vi "Init Edge Detection.vi"(6 "Unsee last word":bool=TRUE, 8 "error in (no error)":errorcluster, 9 "Last output":dbl, 10 "First output":dbl, 11 "RP Transceiver in":refnum<class "RP Transceiver.lvclass">) -> (0 "error out":errorcluster, 3 "RP Transceiver out":refnum<class "RP Transceiver.lvclass">)   [LabVIEW 2016, in "RP Transceiver.lvclass"]
uses:
  RP Transceiver.lvclass
  RP Transceiver.lvclass/RP Transceiver.ctl
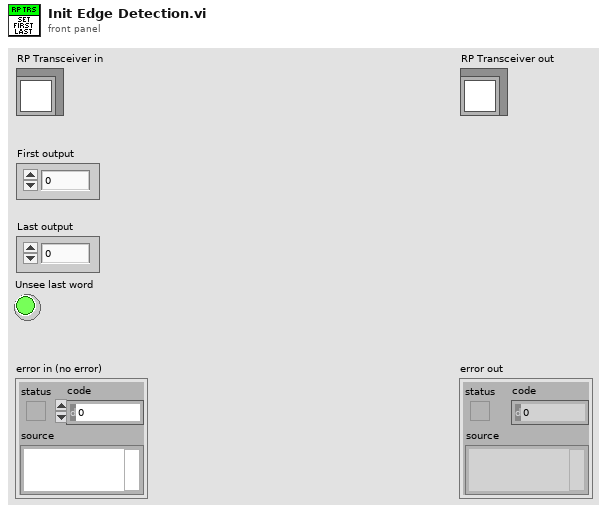
[diagram p1: front panel]
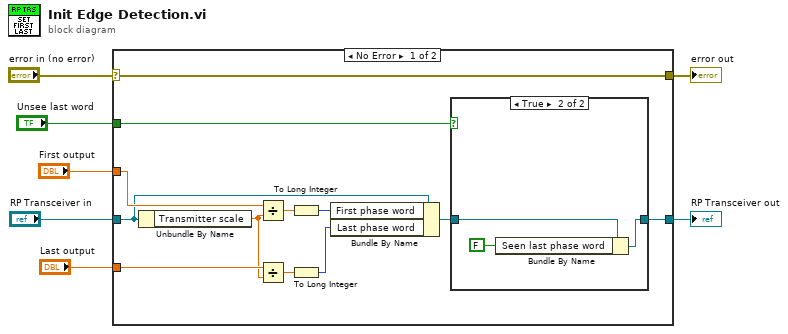
[diagram p0: block diagram]
diagram:
  n1 = case shown="No Error" "error in (no error)" {
    selector: "error in (no error)" -> [w19 w25]
    tunnel: [w19 w25] -> w6
    tunnel: [w9 w24] -> w4
    tunnel: "RP Transceiver in" -> [w11 w24]
    tunnel: "First output" -> [w18 _]
    tunnel: "Last output" -> [w17 _]
    tunnel: "Unsee last word" -> [w8 _]
    frame No Error {
      n2 = Unbundle By Name(w11) -> ("Transmitter scale"=w16:dbl)
      n3 = Divide(x=w18, y=w16) -> (x/y=w15:dbl)
      n4 = Divide(x=w17, y=w16) -> (x/y=w14:dbl)
      n5 = To Long Integer(number=w15) -> (32bit integer=w13:i32)
      n6 = To Long Integer(number=w14) -> (32bit integer=w12:i32)
      n7 = Bundle By Name(cluster=w11, "First phase word"=w13, "Last phase word"=w12) -> (w10:refnum<class "RP Transceiver.lvclass">)
      n8 = case shown="True" w8 {
        tunnel: w10 -> [w20 w23]
        tunnel: [w20 w22] -> w9
        frame False {
        }
        frame True {
          n9 = Bundle By Name(cluster=w23, "Seen last phase word"=FALSE) -> (w22:refnum<class "RP Transceiver.lvclass">)
        }
      }
    }
    frame Error {
    }
  }
  "error out" <- w6
  "RP Transceiver out" <- w4
